vi "SetCommand.vi"(8 "error in (no error)":errorcluster, 10 "Комманда":u8, 11 "StepMotor in":refnum<class "StepMotor.lvclass">) -> (0 "error out":errorcluster, 3 "StepMotor out":refnum<class "StepMotor.lvclass">)   [LabVIEW 2010, in "StepMotor.lvclass"]
doc: "Назначить комманду технологического протокола\nКоманда Краткое описание\n5 Запрос значения парметра из привода (запрос)\n6 Передача от привода текущего значения парметра (ответ)\n7 Установка значения парметра в приводе (запрос)\n17 Запустить программу в ПЛК"
uses:
  StepMotor.lvclass
  StepMotor.lvclass/StepMotor.ctl
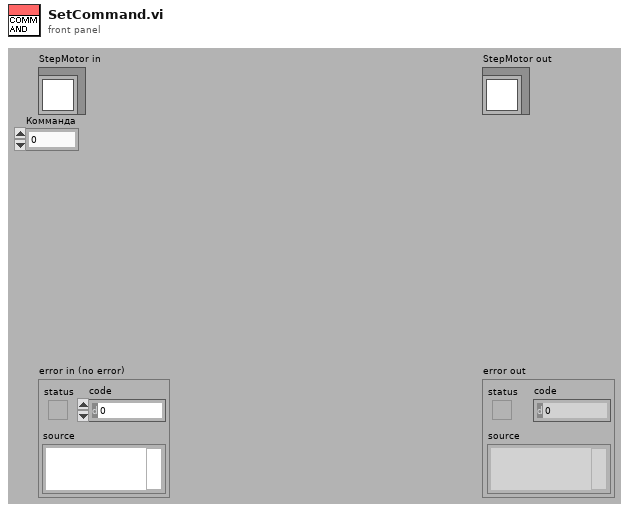
[diagram p1: front panel]
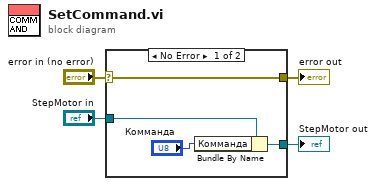
[diagram p0: block diagram]
diagram:
  n1 = case shown="No Error" "error in (no error)" {
    selector: "error in (no error)" -> [w8 w10]
    tunnel: [w8 w10] -> w3
    tunnel: [w6 w9] -> w1
    tunnel: "StepMotor in" -> [w7 w9]
    frame No Error {
      n2 = Bundle By Name(cluster=w7, "Комманда"="Комманда") -> (w6:refnum<class "StepMotor.lvclass">)
    }
    frame Error {
    }
  }
  "error out" <- w3
  "StepMotor out" <- w1
